vi "Ejercicio_15_escritura_digital.vi"() -> ()   [LabVIEW 2020]
panel:
  out "Numeric":dbl
  out "Boolean":bool
  in  "stop":bool
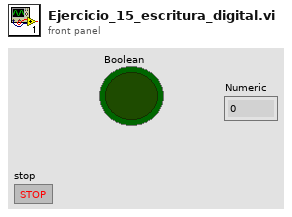
[diagram p1: front panel]
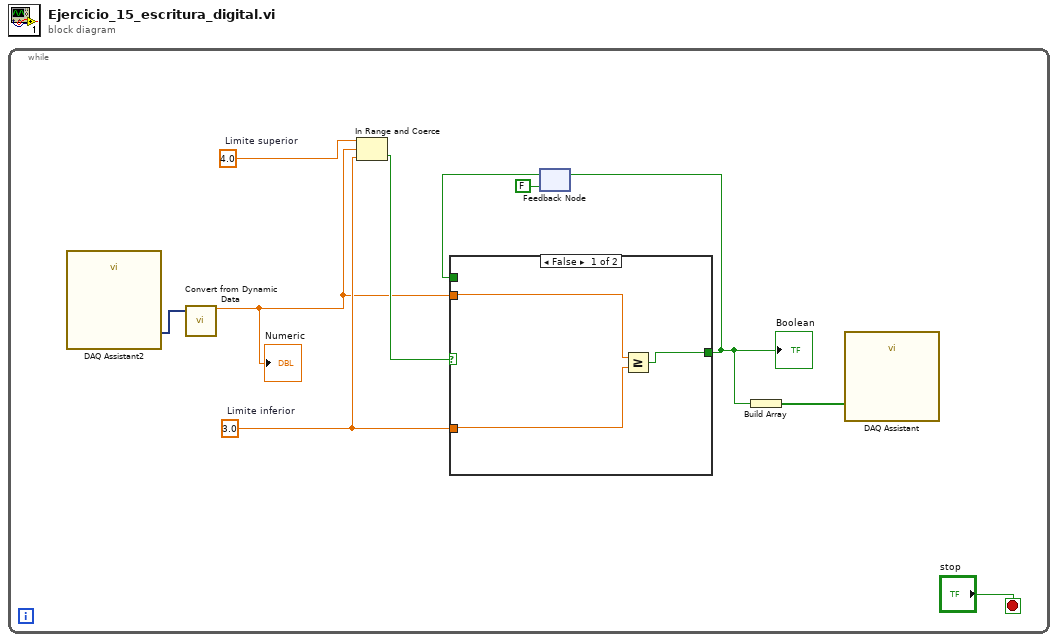
[diagram p0: block diagram]
diagram:
  n1 = while {
    stop <- "stop" stop-if-true
    w6 = 3.0  # Limite inferior
    w9 = 4.0  # Limite superior
    n2 = call "DAQ Assistant2"() -> ("data"=w5:dynamicdata)  [unwired: 17 in, 2 out]
    n3 = call "Convert from Dynamic Data"("Dynamic Data Type"=w5) -> ("Scalar"=w1:dbl)  [unwired: 3 in]
    "Numeric" <- w1
    n4 = In Range and Coerce(upper limit=w9, x=w1, lower limit=w6) -> (In Range?=w4:bool)  [unwired: 1 out]
    n5 = feedback #1(FALSE) -> (w8:bool)
    n6 = case shown="False" w4 {
      tunnel: w1 -> [w13 _]
      tunnel: w6 -> [w12 _]
      tunnel: w8 -> [_ w14]
      tunnel: [w11 w14] -> w3
      frame False {
        n7 = Greater Or Equal?(x=w13, y=w12) -> (x >= y?=w11:bool)
      }
      frame True {
      }
    }
    "Boolean" <- w3
    n8 = feedback-in #1(w3) -> ()
    n9 = Build Array(w3) -> (w2:bool[])
    n10 = call "DAQ Assistant"("data"=w2) -> ()  [unwired: 17 in, 2 out]
  }
